vi "subXMLRemoveTargetNodeSafely.vi"(9 "Target name":string, 10 "Document in":refnum<k20>, 11 "Refnum in":refnum<k20>) -> (0 "error out":errorcluster)   [LabVIEW 2019, in "SolutionBuilder.lvlib" / "SolutionBuilder.lvclass"]
uses:
  SolutionBuilder.lvclass
  <resource>/objmgr/DOMUserDefRef.rc
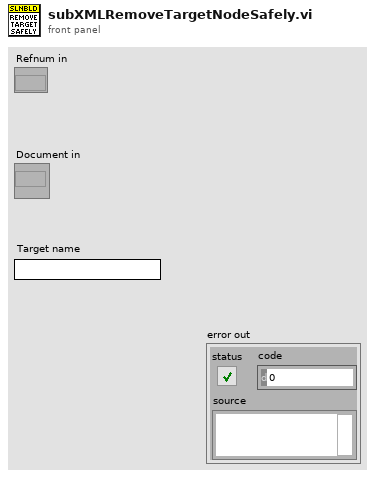
[diagram p1: front panel]
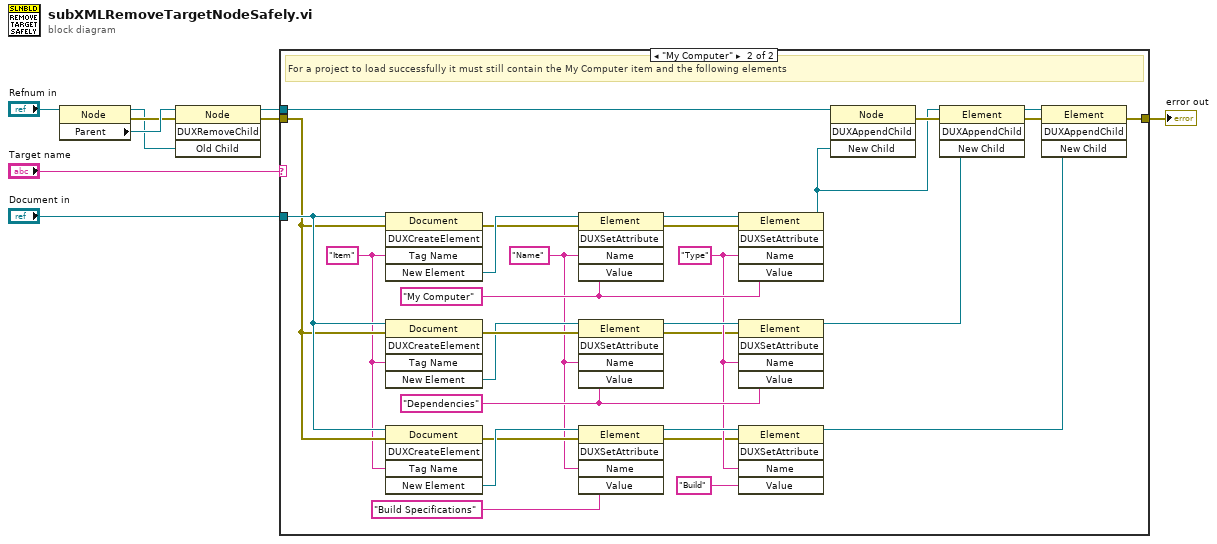
[diagram p0: block diagram]
diagram:
  n1 = property class="Node"(reference="Refnum in") -> (reference out=w4:refnum<k20>, error out=w5:errorcluster, "Parent"=w6:refnum<k20>)  [unwired: 1 in]
  n2 = invoke class="Node" method="DUXRemoveChild"(reference=w6, error in=w5, "Old Child"=w4) -> (reference out=w2:refnum<k20>, error out=w1:errorcluster)  [unwired: 1 in, 2 out]
  n3 = case shown="\"My Computer\"" "Target name" {
    tunnel: w2 -> [_ w21]
    tunnel: [w10 w24] -> w7
    tunnel: "Document in" -> [_ w26]
    tunnel: w1 -> [w10 w18]
    frame Default {
    }
    frame "My Computer" {
      w19 = "Dependencies" ("Value")
      w15 = "Type" ("Name")
      w20 = "My Computer" ("Value")
      w16 = "Name" ("Name")
      w17 = "Item" ("Tag Name")
      # "For a project to load successfully it must still contain the My Computer item and the following elements"
      n4 = invoke class="Document" method="DUXCreateElement"(reference=w26, error in=w18, "Tag Name"=w17) -> (error out=w38:errorcluster, "New Element"=w39:refnum<k20>)  [unwired: 2 in, 3 out]
      n5 = invoke class="Document" method="DUXCreateElement"(reference=w26, error in=w18, "Tag Name"=w17) -> (error out=w35:errorcluster, "New Element"=w34:refnum<k20>)  [unwired: 2 in, 3 out]
      n6 = invoke class="Document" method="DUXCreateElement"(reference=w26, error in=w18, "Tag Name"=w17) -> (error out=w30:errorcluster, "New Element"=w31:refnum<k20>)  [unwired: 2 in, 3 out]
      n7 = invoke class="Element" method="DUXSetAttribute"(reference=w39, error in=w38, "Name"=w16, "Value"=w20) -> (reference out=w37:refnum<k20>, error out=w13:errorcluster)  [unwired: 1 in, 3 out]
      n8 = invoke class="Element" method="DUXSetAttribute"(reference=w34, error in=w35, "Name"=w16, "Value"=w19) -> (reference out=w36:refnum<k20>, error out=w14:errorcluster)  [unwired: 1 in, 3 out]
      n9 = invoke class="Element" method="DUXSetAttribute"(reference=w31, error in=w30, "Name"=w16, "Value"="Build Specifications") -> (reference out=w27:refnum<k20>, error out=w12:errorcluster)  [unwired: 1 in, 3 out]
      n10 = invoke class="Element" method="DUXSetAttribute"(reference=w37, error in=w13, "Name"=w15, "Value"=w20) -> (reference out=w11:refnum<k20>)  [unwired: 1 in, 4 out]
      n11 = invoke class="Element" method="DUXSetAttribute"(reference=w36, error in=w14, "Name"=w15, "Value"=w19) -> (reference out=w33:refnum<k20>)  [unwired: 1 in, 4 out]
      n12 = invoke class="Element" method="DUXSetAttribute"(reference=w27, error in=w12, "Name"=w15, "Value"="Build") -> (reference out=w22:refnum<k20>)  [unwired: 1 in, 4 out]
      n13 = invoke class="Node" method="DUXAppendChild"(reference=w21, "New Child"=w11) -> (error out=w32:errorcluster)  [unwired: 2 in, 3 out]
      n14 = invoke class="Element" method="DUXAppendChild"(reference=w11, error in=w32, "New Child"=w33) -> (reference out=w23:refnum<k20>, error out=w25:errorcluster)  [unwired: 1 in, 2 out]
      n15 = invoke class="Element" method="DUXAppendChild"(reference=w23, error in=w25, "New Child"=w22) -> (error out=w24:errorcluster)  [unwired: 1 in, 3 out]
    }
  }
  "error out" <- w7
